vi "Event handler-Start Stop.vi"(9 "Next State":T1, 11 "UI queue":refnum<queue>) -> (0 "error out":errorcluster, 3 "Queue out":refnum<queue>)   [LabVIEW 2020]
uses:
  Queue/Message Queue/Typedefs/Message Cluster.ctl
  Typedefs/Top level VI states.ctl
  Typedefs/Set Main VI cursor.ctl
  Typedefs/Imaging Protocols enum.ctl
  Typedefs/Start-Stop Enum.ctl
  Global Variables/General Globals.vi
panel:
  # "<---Funct acq fix"
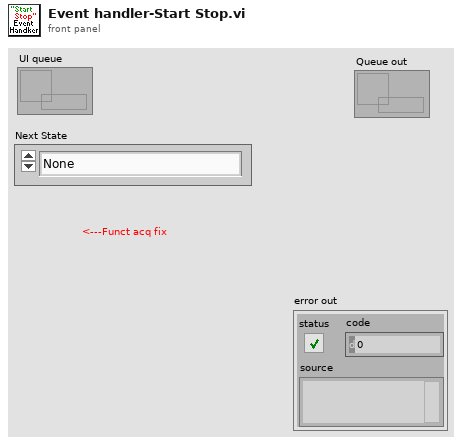
[diagram p1: front panel]
types:
  T1 = typedef "Top level VI states.ctl" = enum16{"None", "Initialise UI", "<STACK PROTOCOL STATES>", "AOL Zstack-START", "AOL Zstack-STOP", "Motor Zstack-START", "Motor Zstack-STOP", "Parameter Sweep-START", "Parameter Sweep-STOP", "<ACQUISITION PROTOCOL STATES> ", "Functional Acquisition-START", "Functional Acquisition-STOP", "Single Plane Acquisition-START", "Single Plane Acquisition-STOP", "Volume Acquisition-START", "Volume Acquisition-STOP", "<LIVE IMAGING PROTOCOL STATES>", "Live Imaging-START", "Live Imaging-STOP", "Live Plane Imaging-START", "Live Plane Imaging-STOP", "Live Volume Imaging-START", "Live Volume Imaging-STOP", "<MOVEMENT CORRECTION PROTOCOL STATES>", "EXIT"}
  T2 = typedef "Set Main VI cursor.ctl" = enum16{"Release busy cursor", "Set busy cursor"}
  T3 = typedef "Imaging Protocols enum.ctl" = enum16{"AOL Z-Stack", "Motor Z Stack", "Parameter Sweep", "Functional Acquisition", "Single Plane Acquisition", "Volume Acquisition", "Live Imaging", "Live Plane Imaging", "Live Volume Imaging"}
  T4 = typedef "Start-Stop Enum.ctl" = enum16{"START", "STOP"}
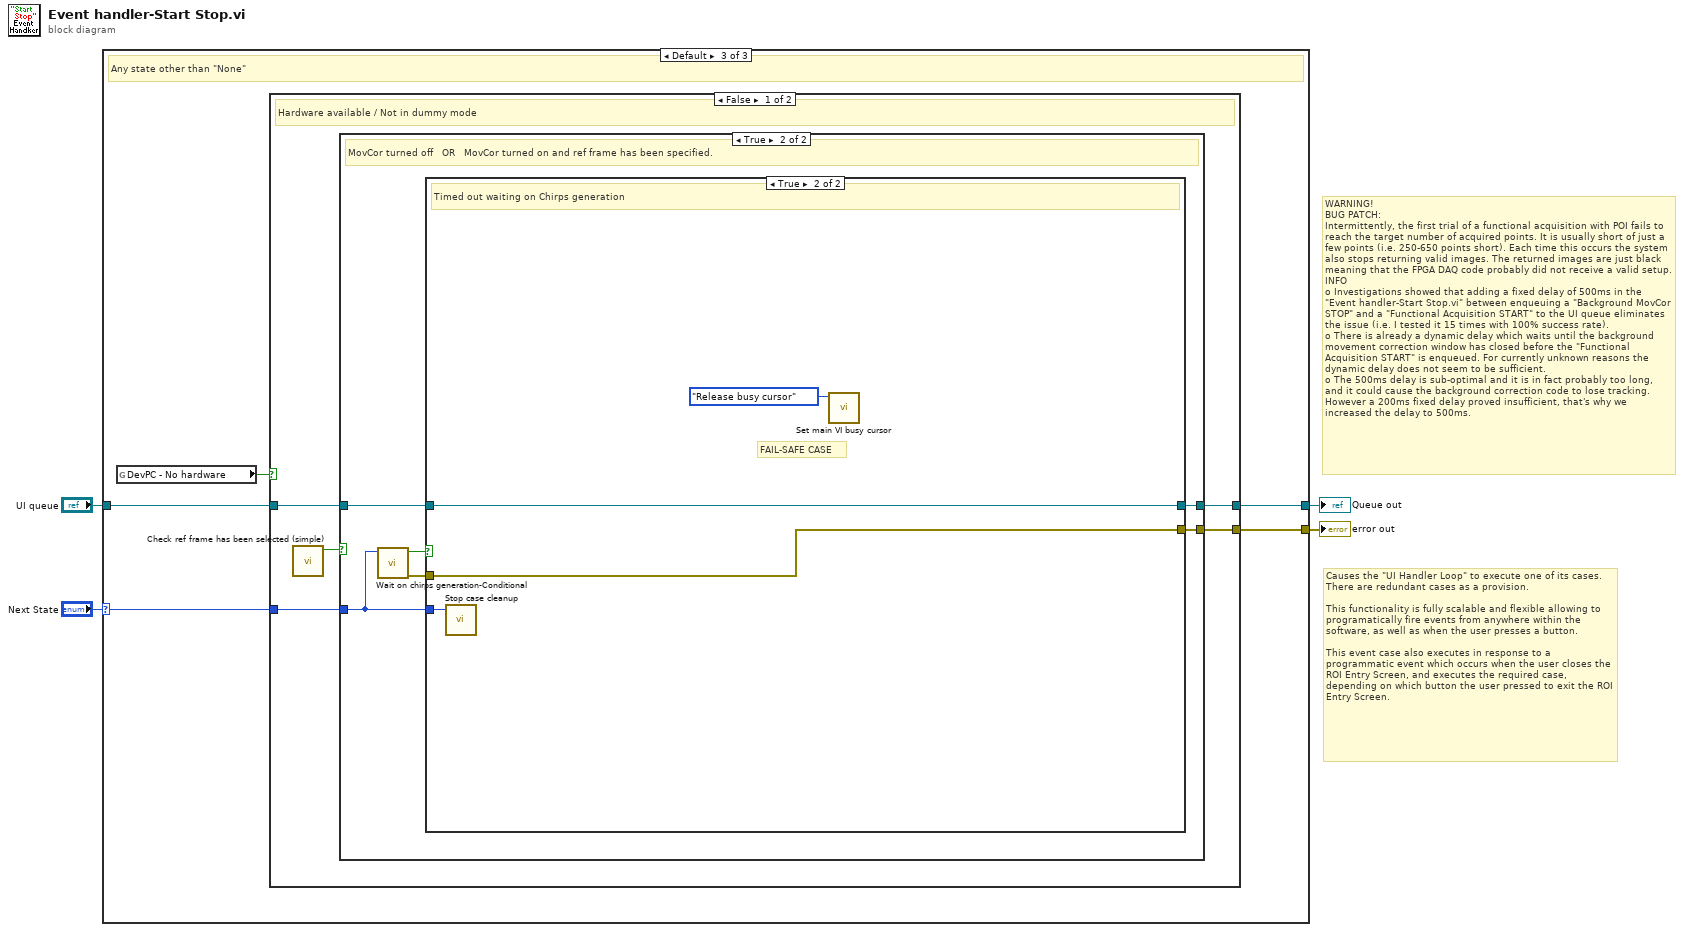
[diagram p0: block diagram]
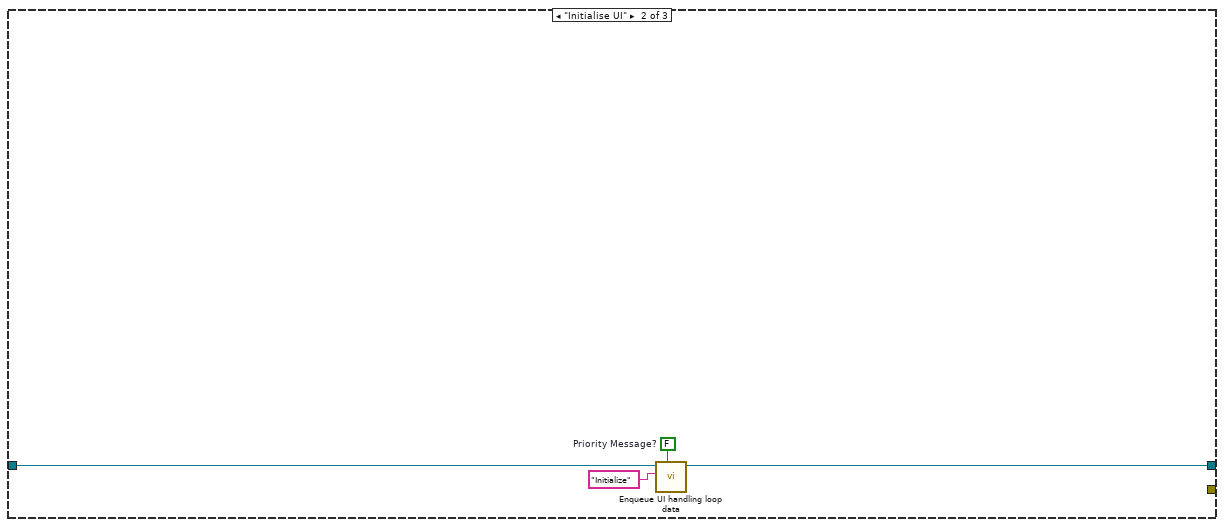
[diagram p3: hidden frame]
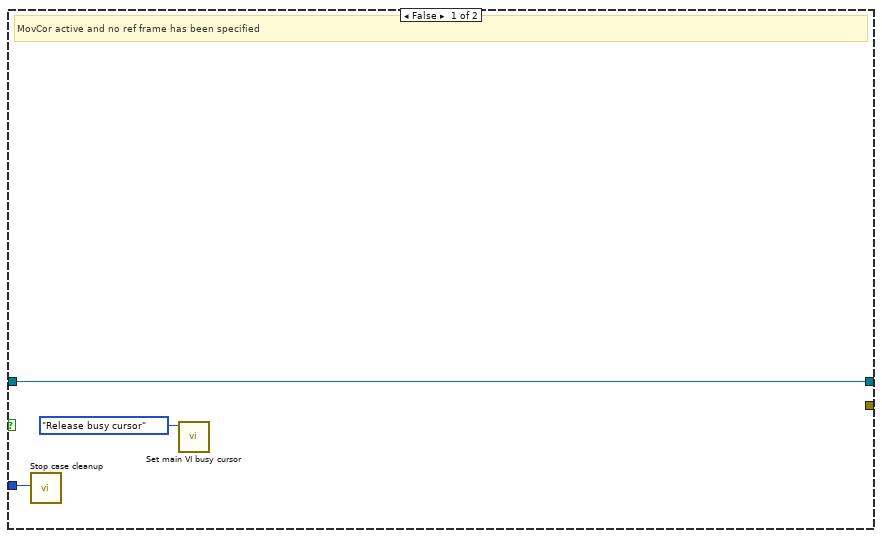
[diagram p4: hidden frame]
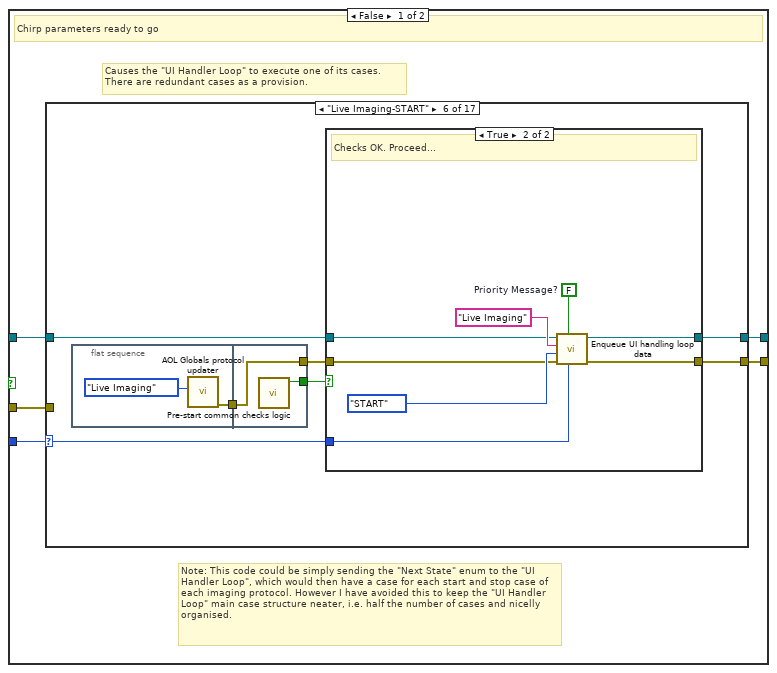
[diagram p5: hidden frame]
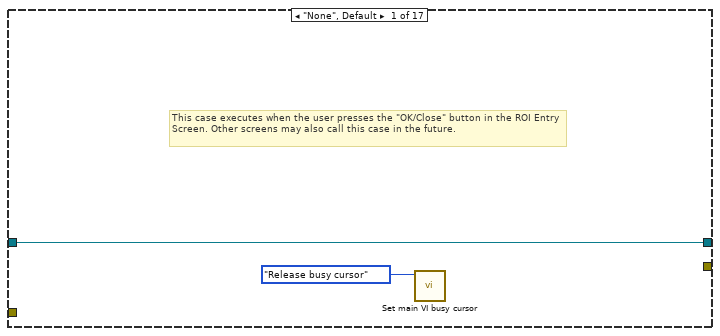
[diagram p6: hidden frame]
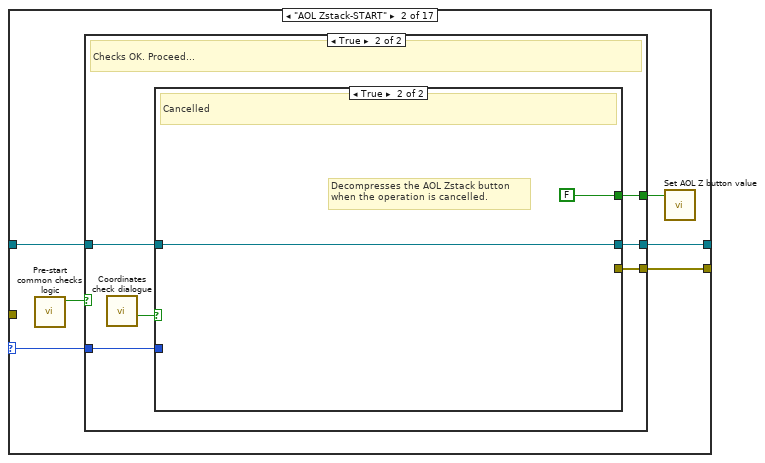
[diagram p7: hidden frame]
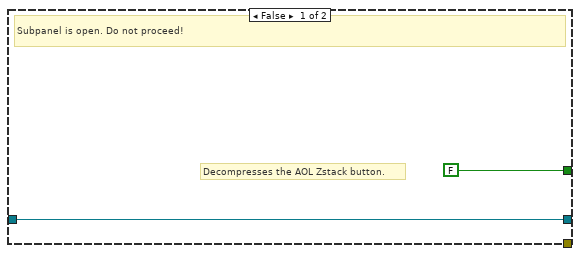
[diagram p8: hidden frame]
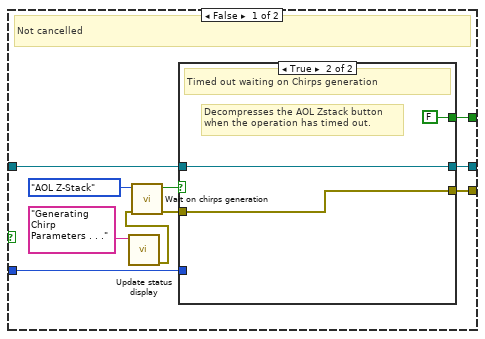
[diagram p9: hidden frame]
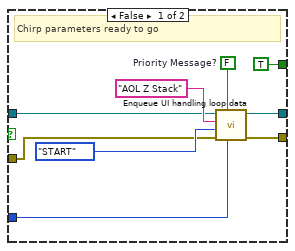
[diagram p10: hidden frame]
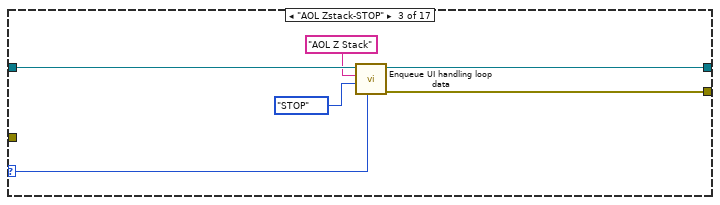
[diagram p11: hidden frame]
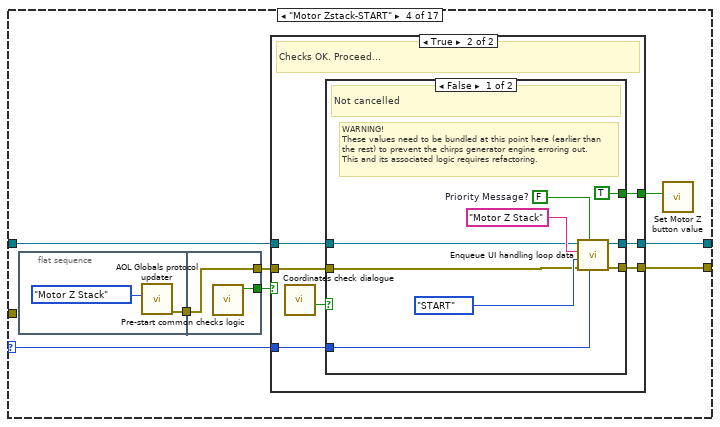
[diagram p12: hidden frame]
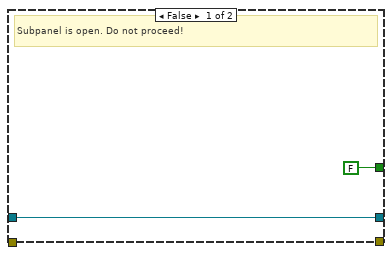
[diagram p13: hidden frame]
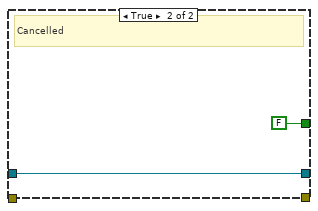
[diagram p14: hidden frame]
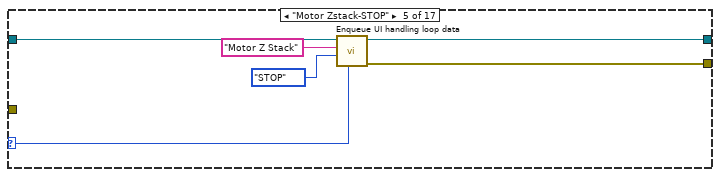
[diagram p15: hidden frame]
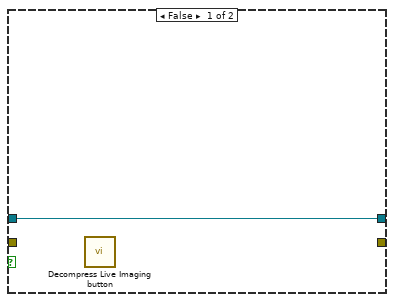
[diagram p16: hidden frame]
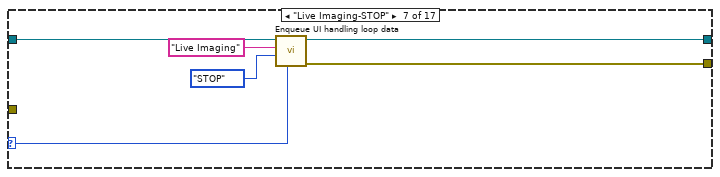
[diagram p17: hidden frame]
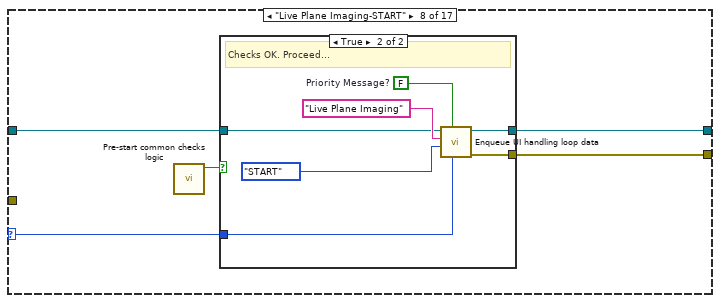
[diagram p18: hidden frame]
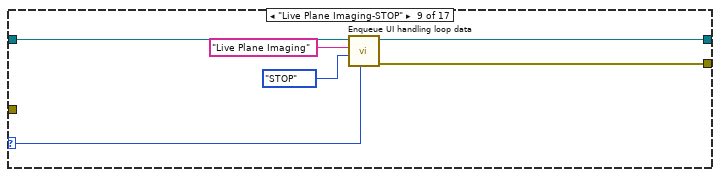
[diagram p20: hidden frame]
diagram:
  # "Causes the \"UI Handler Loop\" to execute one of its cases. There are redundant cases as a provision.\n\nThis functionality is fully scalable and flexible allowing to programatically fire events from anywhere within the software, as well as when the user presses a button.\n\nThis event case also executes in response to a programmatic event which occurs when the user closes the ROI Entry Screen, and executes the required case, depending on which button the user pressed to exit the ROI Entry Screen."
  # "WARNING!\nBUG PATCH: \nIntermittently, the first trial of a functional acquisition with POI fails to reach the target number of acquired points. It is usually short of just a few points (i.e. 250-650 points short). Each time this occurs the system also stops returning valid images. The returned images are just black meaning that the FPGA DAQ code probably did not receive a valid setup.\nINFO\no\tInvestigations showed that adding a fixed delay of 500ms in the \"Event handler-Start Stop.vi\" between enqueuing a \"Background MovCor STOP\" and a \"Functional Acquisition START\" to the UI queue eliminates the issue (i.e. I tested it 15 times with 100% success rate).\no\tThere is already a dynamic delay which waits until the background movement correction window has closed before the \"Functional Acquisition START\" is enqueued. For currently unknown reasons the dynamic delay does not seem to be sufficient.\no\tThe 500ms delay is sub-optimal and it is in fact probably too long, and it could cause the background correction code to lose tracking. However a 200ms fixed delay proved insufficient, that's why we increased the delay to 500ms."
  n1 = case shown="Default" "Next State" {
    selector: "Next State" -> [_ _ w11]
    tunnel: "UI queue" -> [w5 w9 w14]
    tunnel: [_ _ w13] -> w3
    tunnel: [w5 w8 w12] -> w2
    frame "None" {
    }
    frame "Initialise UI" {
      w6 = FALSE  # Priority Message?
      n2 = call "Enqueue UI handling loop data.vi"("Priority Message? (T)"=w6, "Message"="Initialize", "Queue in"=w9) -> ("Queue out"=w8:refnum<queue>)  [unwired: 7 in, 1 out]
    }
    frame Default {
      # "Any state other than \"None\""
      n3 = global read "General Globals.vi" "DevPC - No hardware"() -> (w10:bool)
      n4 = case shown="False" w10 {
        tunnel: w14 -> [w19 w249]
        tunnel: [w18 _] -> w13
        tunnel: [w17 w249] -> w12
        tunnel: w11 -> [w15 w248]
        frame False {
          # "Hardware available / Not in dummy mode"
          n5 = call "Check ref frame has been selected (simple).vi"() -> ("Proceed / Reference frame has been selected"=w16:bool)  [unwired: 10 in, 1 out]
          n6 = case shown="True" w16 {
            tunnel: w19 -> [w22 w28]
            tunnel: [_ w27] -> w18
            tunnel: [w22 w26] -> w17
            tunnel: w15 -> [w21 w25]
            frame False {
              # "MovCor active and no ref frame has been specified"
              n7 = call "Stop case cleanup.vi"("Next State"=w21) -> ()  [unwired: 11 in]
              n8 = call "Set main VI busy cursor.vi"("Main VI's cursor"=Set_Main_VI_cursor."Release busy cursor") -> ()  [unwired: 10 in, 1 out]
            }
            frame True {
              # "MovCor turned off   OR   MovCor turned on and ref frame has been specified."
              n9 = call "Wait on chirps generation-Conditional.vi"("Next State"=w25) -> ("error out"=w23:errorcluster, "Timed out waiting on Chirps generation"=w24:bool)  [unwired: 9 in]
              n10 = case shown="True" w24 {
                tunnel: w28 -> [w33 w247]
                tunnel: w25 -> [w32 w244]
                tunnel: [w31 w245] -> w27
                tunnel: [w30 w247] -> w26
                tunnel: w23 -> [w29 w245]
                frame False {
                  # "Note: This code could be simply sending the \"Next State\" enum to the \"UI Handler Loop\", which would then have a case for each start and stop case of each imaging protocol. However I have avoided this to keep the \"UI Handler Loop\" main case structure neater, i.e. half the number of cases and nicelly organised."
                  # "Causes the \"UI Handler Loop\" to execute one of its cases.\nThere are redundant cases as a provision."
                  # "Chirp parameters ready to go"
                  n11 = case shown="\"Live Imaging-START\"" w32 {
                    selector: w32 -> [_ w37 w76 w85 w114 w123 w141 w147 w160 w166 w180 w185 w202 w208 w223 w227 w241]
                    tunnel: w33 -> [w35 w41 w79 w87 w116 w121 w142 w146 w162 w164 w181 w187 w204 w210 w224 w229 w242]
                    tunnel: [_ w40 w78 w86 w112 w124 w139 w148 w157 w167 w176 w186 w200 w209 w219 w228 w238] -> w31
                    tunnel: [w35 w39 w75 w84 w113 w122 w140 w145 w158 w165 w177 w184 w201 w207 w220 w226 w239] -> w30
                    tunnel: w29 -> [_ _ _ _ _ _ _ _ _ _ _ _ _ _ _ _ _]
                    frame "None", Default {
                      # "This case executes when the user presses the \"OK/Close\" button in the ROI Entry Screen. Other screens may also call this case in the future."
                      n12 = call "Set main VI busy cursor.vi"("Main VI's cursor"=Set_Main_VI_cursor."Release busy cursor") -> ()  [unwired: 10 in, 1 out]
                    }
                    frame "AOL Zstack-START" {
                      n13 = call "Pre-start common checks logic.vi"() -> ("Proceed"=w38:bool)  [unwired: 11 in]
                      n14 = case shown="True" w38 {
                        tunnel: w41 -> [w43 w49]
                        tunnel: [_ w48] -> w40
                        tunnel: w37 -> [_ w47]
                        tunnel: [w43 w46] -> w39
                        tunnel: [FALSE ("Value") w44] -> w36
                        frame False {
                          # "Decompresses the AOL Zstack button."
                          # "Subpanel is open. Do not proceed!"
                        }
                        frame True {
                          # "Checks OK. Proceed..."
                          n15 = call "Coordinates check dialogue.vi"() -> ("Cancelled"=w45:bool)  [unwired: 11 in]
                          n16 = case shown="True" w45 {
                            tunnel: w49 -> [w54 w73]
                            tunnel: [w59 _] -> w48
                            tunnel: w47 -> [w57 _]
                            tunnel: [w58 w73] -> w46
                            tunnel: [w50 FALSE ("Value")] -> w44
                            frame False {
                              # "Not cancelled"
                              n17 = call "Update status display.vi"("Acquiring and Logging..."="Generating Chirp Parameters . . .") -> ("error out"=w52:errorcluster)  [unwired: 10 in]
                              n18 = call "Wait on chirps generation.vi"("error in (no error)"=w52, "Imaging Protocol"=Imaging_Protocols_enum."AOL Z-Stack") -> ("error out"=w51:errorcluster, "Timed out waiting on Chirps generation"=w55:bool)  [unwired: 8 in]
                              n19 = case shown="True" w55 {
                                tunnel: [w68 w70] -> w59
                                tunnel: w54 -> [w61 w71]
                                tunnel: [w66 w71] -> w58
                                tunnel: w57 -> [w63 _]
                                tunnel: w51 -> [w60 w70]
                                tunnel: [TRUE ("Value") FALSE ("Value")] -> w50
                                frame False {
                                w64 = FALSE  # Priority Message?
                                # "Chirp parameters ready to go"
                                n20 = call "Enqueue UI handling loop data.vi"("Next State"=w63, "Priority Message? (T)"=w64, "error in (no error)"=w60, "Start/Stop"=Start-Stop_Enum."START", "Message"="AOL Z Stack", "Queue in"=w61) -> ("error out"=w68:errorcluster, "Queue out"=w66:refnum<queue>)  [unwired: 4 in]
                                }
                                frame True {
                                # "Decompresses the AOL Zstack button\nwhen the operation has timed out."
                                # "Timed out waiting on Chirps generation"
                                }
                              }
                            }
                            frame True {
                              # "Decompresses the AOL Zstack button\nwhen the operation is cancelled."
                              # "Cancelled"
                            }
                          }
                        }
                      }
                      n21 = call "Set AOL Z button value.vi"("AOL Z button's new value"=w36) -> ()  [unwired: 10 in, 1 out]
                    }
                    frame "AOL Zstack-STOP" {
                      n22 = call "Enqueue UI handling loop data.vi"("Next State"=w76, "Start/Stop"=Start-Stop_Enum."STOP", "Message"="AOL Z Stack", "Queue in"=w79) -> ("error out"=w78:errorcluster, "Queue out"=w75:refnum<queue>)  [unwired: 6 in]
                    }
                    frame "Motor Zstack-START" {
                      n23 = flat-sequence {
                        tunnel: [w88] -> w83
                        tunnel: [w91] -> w82
                        tunnel: [w90] -> w81
                        tunnel: w83 -> [w90]
                        frame #0 {
                          n24 = call "AOL Globals protocol updater.vi"("Imaging Mode"=Imaging_Protocols_enum."Motor Z Stack") -> ("error out"=w88:errorcluster)  [unwired: 10 in]
                        }
                        frame #1 {
                          n25 = call "Pre-start common checks logic.vi"() -> ("Proceed"=w91:bool)  [unwired: 11 in]
                        }
                      }
                      n26 = case shown="True" w82 {
                        tunnel: w87 -> [w93 w100]
                        tunnel: [_ w99] -> w86
                        tunnel: w85 -> [_ w98]
                        tunnel: [w93 w97] -> w84
                        tunnel: w81 -> [_ w95]
                        tunnel: [FALSE w94] -> w80
                        frame False {
                          # "Subpanel is open. Do not proceed!"
                        }
                        frame True {
                          # "Checks OK. Proceed..."
                          n27 = call "Coordinates check dialogue.vi"() -> ("Cancelled"=w96:bool)  [unwired: 11 in]
                          n28 = case shown="False" w96 {
                            tunnel: w100 -> [w102 w111]
                            tunnel: [w108 _] -> w99
                            tunnel: w98 -> [w104 _]
                            tunnel: [w106 w111] -> w97
                            tunnel: w95 -> [w101 _]
                            tunnel: [TRUE FALSE] -> w94
                            frame False {
                              w105 = FALSE  # Priority Message?
                              # "WARNING!\nThese values need to be bundled at this point here (earlier than the rest) to prevent the chirps generator engine erroring out.\nThis and its associated logic requires refactoring."
                              # "Not cancelled"
                              n29 = call "Enqueue UI handling loop data.vi"("Next State"=w104, "Priority Message? (T)"=w105, "error in (no error)"=w101, "Start/Stop"=Start-Stop_Enum."START", "Message"="Motor Z Stack", "Queue in"=w102) -> ("error out"=w108:errorcluster, "Queue out"=w106:refnum<queue>)  [unwired: 4 in]
                            }
                            frame True {
                              # "Cancelled"
                            }
                          }
                        }
                      }
                      n30 = call "Set Motor Z button value.vi"("Motor Z button's new value"=w80) -> ()  [unwired: 10 in, 1 out]
                    }
                    frame "Motor Zstack-STOP" {
                      n31 = call "Enqueue UI handling loop data.vi"("Next State"=w114, "Start/Stop"=Start-Stop_Enum."STOP", "Message"="Motor Z Stack", "Queue in"=w116) -> ("error out"=w112:errorcluster, "Queue out"=w113:refnum<queue>)  [unwired: 6 in]
                    }
                    frame "Live Imaging-START" {
                      n32 = flat-sequence {
                        tunnel: [w125] -> w118
                        tunnel: [w128] -> w120
                        tunnel: [w127] -> w119
                        tunnel: w118 -> [w127]
                        frame #0 {
                          n33 = call "AOL Globals protocol updater.vi"("Imaging Mode"=Imaging_Protocols_enum."Live Imaging") -> ("error out"=w125:errorcluster)  [unwired: 10 in]
                        }
                        frame #1 {
                          n34 = call "Pre-start common checks logic.vi"() -> ("Proceed"=w128:bool)  [unwired: 11 in]
                        }
                      }
                      n35 = case shown="True" w120 {
                        tunnel: [_ w136] -> w124
                        tunnel: w123 -> [_ w132]
                        tunnel: [w129 w135] -> w122
                        tunnel: w121 -> [w129 w131]
                        tunnel: w119 -> [_ w130]
                        frame False {
                          n36 = call "Decompress Live Imaging button.vi"() -> ()  [unwired: 12 in]
                        }
                        frame True {
                          w133 = FALSE  # Priority Message?
                          # "Checks OK. Proceed..."
                          n37 = call "Enqueue UI handling loop data.vi"("Next State"=w132, "Priority Message? (T)"=w133, "error in (no error)"=w130, "Start/Stop"=Start-Stop_Enum."START", "Message"="Live Imaging", "Queue in"=w131) -> ("error out"=w136:errorcluster, "Queue out"=w135:refnum<queue>)  [unwired: 4 in]
                        }
                      }
                    }
                    frame "Live Imaging-STOP" {
                      n38 = call "Enqueue UI handling loop data.vi"("Next State"=w141, "Start/Stop"=Start-Stop_Enum."STOP", "Message"="Live Imaging", "Queue in"=w142) -> ("error out"=w139:errorcluster, "Queue out"=w140:refnum<queue>)  [unwired: 6 in]
                    }
                    frame "Live Plane Imaging-START" {
                      n39 = call "Pre-start common checks logic.vi"() -> ("Proceed"=w144:bool)  [unwired: 11 in]
                      n40 = case shown="True" w144 {
                        tunnel: [_ w156] -> w148
                        tunnel: w147 -> [_ w150]
                        tunnel: w146 -> [w149 w151]
                        tunnel: [w149 w154] -> w145
                        frame False {
                        }
                        frame True {
                          w153 = FALSE  # Priority Message?
                          # "Checks OK. Proceed..."
                          n41 = call "Enqueue UI handling loop data.vi"("Next State"=w150, "Priority Message? (T)"=w153, "Start/Stop"=Start-Stop_Enum."START", "Message"="Live Plane Imaging", "Queue in"=w151) -> ("error out"=w156:errorcluster, "Queue out"=w154:refnum<queue>)  [unwired: 5 in]
                        }
                      }
                    }
                    frame "Live Plane Imaging-STOP" {
                      n42 = call "Enqueue UI handling loop data.vi"("Next State"=w160, "Start/Stop"=Start-Stop_Enum."STOP", "Message"="Live Plane Imaging", "Queue in"=w162) -> ("error out"=w157:errorcluster, "Queue out"=w158:refnum<queue>)  [unwired: 6 in]
                    }
                    frame "Live Volume Imaging-START" {
                      n43 = call "Pre-start common checks logic.vi"() -> ("Proceed"=w163:bool)  [unwired: 11 in]
                      n44 = case shown="True" w163 {
                        tunnel: [_ w175] -> w167
                        tunnel: w166 -> [_ w170]
                        tunnel: [w168 w173] -> w165
                        tunnel: w164 -> [w168 w169]
                        frame False {
                        }
                        frame True {
                          w171 = FALSE  # Priority Message?
                          # "Checks OK. Proceed..."
                          n45 = call "Enqueue UI handling loop data.vi"("Next State"=w170, "Priority Message? (T)"=w171, "Start/Stop"=Start-Stop_Enum."START", "Message"="Live volume imaging", "Queue in"=w169) -> ("error out"=w175:errorcluster, "Queue out"=w173:refnum<queue>)  [unwired: 5 in]
                        }
                      }
                    }
                    frame "Live Volume Imaging-STOP" {
                      n46 = call "Enqueue UI handling loop data.vi"("Next State"=w180, "Start/Stop"=Start-Stop_Enum."STOP", "Message"="Live volume imaging", "Queue in"=w181) -> ("error out"=w176:errorcluster, "Queue out"=w177:refnum<queue>)  [unwired: 6 in]
                    }
                    frame "Functional Acquisition-START" {
                      n47 = call "Pre-start common checks logic.vi"() -> ("Proceed"=w182:bool)  [unwired: 11 in]
                      n48 = case shown="True" w182 {
                        tunnel: [FALSE ("Proceed") w189] -> w183
                        frame False {
                        }
                        frame True {
                          n49 = call "Funct acq pre-checks.vi"() -> ("Proceed"=w189:bool)  [unwired: 11 in]
                        }
                      }
                      n50 = case shown="True" w183 {
                        tunnel: w187 -> [w191 w192]
                        tunnel: [_ w199] -> w186
                        tunnel: w185 -> [_ w196]
                        tunnel: [w191 w197] -> w184
                        frame False {
                          # "Fail-safe logic.\nReleases the functional acquisition button if pressed."
                          # "Cannot be allowed to start"
                          n51 = call "Set Funct Acq button value.vi"("Functional Acquisition button's new value"=FALSE ("Value")) -> ()  [unwired: 10 in, 1 out]
                        }
                        frame True {
                          w194 = FALSE  # Priority Message?
                          w198 = Start-Stop_Enum."START"  # Main protocol
                          # "Allowed to start"
                          n52 = call "Set Funct Acq button value.vi"("Functional Acquisition button's new value"=TRUE ("Value")) -> ()  [unwired: 10 in, 1 out]
                          n53 = call "Enqueue UI handling loop data.vi"("Next State"=w196, "Priority Message? (T)"=w194, "Start/Stop"=w198, "Message"="Functional Acquisition", "Queue in"=w192) -> ("error out"=w199:errorcluster, "Queue out"=w197:refnum<queue>)  [unwired: 5 in]
                        }
                      }
                    }
                    frame "Functional Acquisition-STOP" {
                      # "Simply causes the UI to be re-enabled as soon as the functional data has been post processed (and displayed in the viewer where applicable)."
                      n54 = call "Enqueue UI handling loop data.vi"("Next State"=w202, "Start/Stop"=Start-Stop_Enum."STOP", "Message"="Functional Acquisition", "Queue in"=w204) -> ("error out"=w200:errorcluster, "Queue out"=w201:refnum<queue>)  [unwired: 6 in]
                    }
                    frame "Single Plane Acquisition-START" {
                      n55 = call "Pre-start common checks logic.vi"() -> ("Proceed"=w206:bool)  [unwired: 11 in]
                      n56 = case shown="True" w206 {
                        tunnel: w210 -> [w211 w212]
                        tunnel: [_ w218] -> w209
                        tunnel: w208 -> [_ w213]
                        tunnel: [w211 w217] -> w207
                        frame False {
                          # "ADD CODE HERE TO DECOMPRESS\nTHE FP BUTTON IF ONE IS ADDED LATER FOR THIS PROTOCOL."
                          # "May not start / HDD space low"
                        }
                        frame True {
                          w214 = FALSE  # Priority Message?
                          # "Allowed to start"
                          n57 = call "Enqueue UI handling loop data.vi"("Next State"=w213, "Priority Message? (T)"=w214, "Start/Stop"=Start-Stop_Enum."START", "Message"="Single Plane Acquisition", "Queue in"=w212) -> ("error out"=w218:errorcluster, "Queue out"=w217:refnum<queue>)  [unwired: 5 in]
                        }
                      }
                    }
                    frame "Single Plane Acquisition-STOP" {
                      n58 = call "Enqueue UI handling loop data.vi"("Next State"=w223, "Start/Stop"=Start-Stop_Enum."STOP", "Message"="Single Plane Acquisition", "Queue in"=w224) -> ("error out"=w219:errorcluster, "Queue out"=w220:refnum<queue>)  [unwired: 6 in]
                    }
                    frame "Volume Acquisition-START" {
                      n59 = call "Pre-start common checks logic.vi"() -> ("Proceed"=w225:bool)  [unwired: 11 in]
                      n60 = case shown="True" w225 {
                        tunnel: w229 -> [w230 w231]
                        tunnel: [_ w237] -> w228
                        tunnel: w227 -> [_ w232]
                        tunnel: [w230 w234] -> w226
                        frame False {
                          # "ADD CODE HERE TO DECOMPRESS\nTHE FP BUTTON IF ONE IS ADDED LATER FOR THIS PROTOCOL."
                          # "May not start / HDD space low"
                        }
                        frame True {
                          w233 = FALSE  # Priority Message?
                          # "Allowed to start"
                          n61 = call "Enqueue UI handling loop data.vi"("Next State"=w232, "Priority Message? (T)"=w233, "Start/Stop"=Start-Stop_Enum."START", "Message"="Volume acquisition", "Queue in"=w231) -> ("error out"=w237:errorcluster, "Queue out"=w234:refnum<queue>)  [unwired: 5 in]
                        }
                      }
                    }
                    frame "Volume Acquisition-STOP" {
                      n62 = call "Enqueue UI handling loop data.vi"("Next State"=w241, "Start/Stop"=Start-Stop_Enum."STOP", "Message"="Volume acquisition", "Queue in"=w242) -> ("error out"=w238:errorcluster, "Queue out"=w239:refnum<queue>)  [unwired: 6 in]
                    }
                  }
                }
                frame True {
                  # "FAIL-SAFE CASE"
                  # "Timed out waiting on Chirps generation"
                  n63 = call "Stop case cleanup.vi"("Next State"=w244) -> ()  [unwired: 11 in]
                  n64 = call "Set main VI busy cursor.vi"("Main VI's cursor"=Set_Main_VI_cursor."Release busy cursor") -> ()  [unwired: 10 in, 1 out]
                }
              }
            }
          }
        }
        frame True {
          # "Prevents execution start of all main functions when the hardware is unavailable (i.e. when dummy mode is active)"
          # "Dummy mode"
          n65 = flat-sequence {
            tunnel: w248 -> [w250]
            frame #0 {
              n66 = call "Set main VI busy cursor.vi"("Main VI's cursor"=Set_Main_VI_cursor."Release busy cursor") -> ()  [unwired: 10 in, 1 out]
              n67 = call "Stop case cleanup.vi"("Next State"=w250) -> ()  [unwired: 11 in]
            }
            frame #1 {
              n68 = call "Message Window.vi"("Message string"="This function cannot be used when the hardware is unavailable.") -> ()  [unwired: 10 in, 1 out]
            }
          }
        }
      }
    }
  }
  "error out" <- w3
  "Queue out" <- w2
